vi "Write.vi"(8 "error in (no error)":errorcluster, 10 "Write Buffer":string, 11 "VISA resource name":refnum<visa-resource-name>) -> (0 "error out":errorcluster, 3 "VISA resource name out":refnum<visa-resource-name>)   [LabVIEW 2015, in "Fluke 289.lvlib"]
doc: "Replaces LabVIEW VISA Write. For each write command, a carriage return constant appens to the command, and an acknowledge value is returned. The value indicates correct or incorrect operation."
uses:
  <instrlib>/Fluke 289/Fluke 289.lvlib
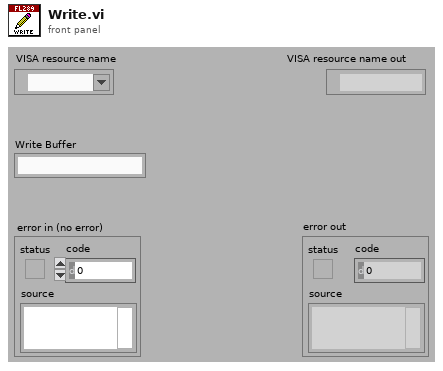
[diagram p1: front panel]
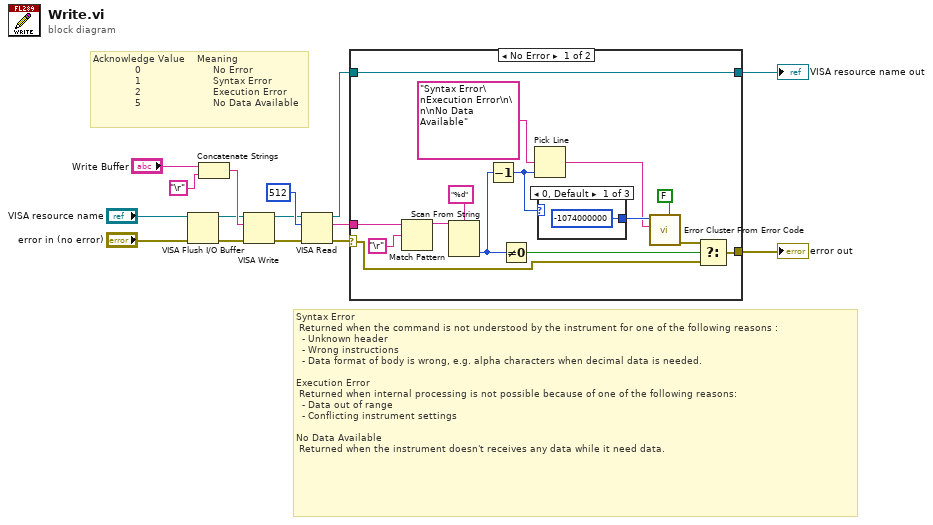
[diagram p0: block diagram]
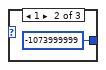
[diagram p2: hidden frame]
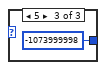
[diagram p3: hidden frame]
diagram:
  # "Acknowledge Value    Meaning\n              0                        No Error\n              1                        Syntax Error\n              2                        Execution Error\n              5                        No Data Available"
  # "Syntax Error\n Returned when the command is not understood by the instrument for one of the following reasons :\n  - Unknown header\n  - Wrong instructions\n  - Data format of body is wrong, e.g. alpha characters when decimal data is needed.\n\nExecution Error\n Returned when internal processing is not possible because of one of the following reasons:\n  - Data out of range\n  - Conflicting instrument settings\n\nNo Data Available\n Returned when the instrument doesn't receives any data while it need data."
  n1 = VISA Flush I/O Buffer(VISA resource name="VISA resource name", error in (no error)="error in (no error)") -> (VISA resource name out=w12:refnum<visa-resource-name>, error out=w11:errorcluster)  [unwired: 1 in]
  n2 = Concatenate Strings("Write Buffer", "\r") -> (w13:string)
  n3 = VISA Write(VISA resource name=w12, write buffer=w13, error in (no error)=w11) -> (VISA resource name out=w5:refnum<visa-resource-name>, error out=w6:errorcluster)  [unwired: 1 out]
  n4 = VISA Read(VISA resource name=w5, byte count=u32 512, error in (no error)=w6) -> (VISA resource name out=w9:refnum<visa-resource-name>, read buffer=w8:string, error out=w7:errorcluster)  [unwired: 1 out]
  n5 = case shown="No Error" w7 {
    selector: w7 -> [w25 w35]
    tunnel: w8 -> [w30 _]
    tunnel: w9 -> [w16 w34]
    tunnel: [w24 w35] -> w2
    tunnel: [w16 w34] -> w1
    frame No Error {
      n6 = Match Pattern(string=w30, regular expression="\r") -> (before substring=w28:string)  [unwired: 1 in, 3 out]
      n7 = Scan From String(format string="%d", input string=w28) -> (output 1=w21:i32)  [unwired: 3 in, 3 out]
      n8 = Decrement(x=w21) -> (x-1=w19:i32)
      n9 = Not Equal To 0?(x=w21) -> (x != 0?=w26:bool)
      n10 = Pick Line(multi-line string="Syntax Error\nExecution Error\n\n\nNo Data Available", line index=w19) -> (output string=w17:string)  [unwired: 1 in]
      n11 = case shown="0, Default" w19 {
        tunnel: [-1074000000 -1073999999 -1073999998] -> w18
        frame 0, Default {
        }
        frame 1 {
        }
        frame 5 {
        }
      }
      n12 = call <vilib>:"Error Cluster From Error Code.vi"("is warning? (False)"=FALSE, "error message (\"\")"=w17, "error code (0)"=w18) -> ("error out"=w22:errorcluster)  [unwired: 6 in]
      n13 = Select(t=w22, s=w26, f=w25) -> (s? t:f=w24:errorcluster)
    }
    frame Error {
    }
  }
  "error out" <- w2
  "VISA resource name out" <- w1
